vi "OUTPUT(Advanced).vi"(8 "Error In":errorcluster, 11 "VISA resource name":refnum<visa-resource-name>) -> (0 "Error Out":errorcluster, 3 "VISA resource name out":refnum<visa-resource-name>)   [LabVIEW 2013]
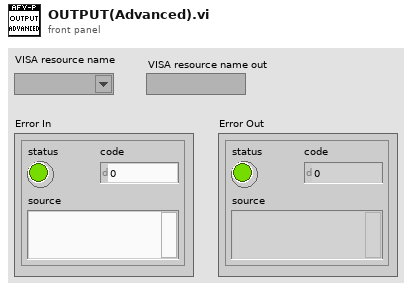
[diagram p1: front panel]
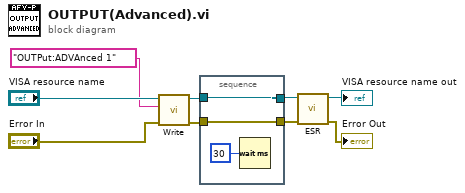
[diagram p0: block diagram]
diagram:
  n1 = call "Write.vi"("Error In"="Error In", "Write Buffer"="OUTPut:ADVAnced 1", "VISA resource name"="VISA resource name") -> ("Error Out"=w1:errorcluster, "VISA resource name out"=w2:refnum<visa-resource-name>)  [unwired: 7 in]
  n2 = stacked-sequence {
    tunnel: [w11] -> w6
    tunnel: w2 -> [w11]
    tunnel: [w10] -> w5
    tunnel: w1 -> [w10]
    frame #0 {
      n3 = Wait (ms)(milliseconds to wait=u32 30) -> ()  [unwired: 1 out]
    }
  }
  n4 = call "ESR.vi"("Error In"=w5, "VISA resource name"=w6) -> ("Error Out"=→"Error Out":errorcluster, "VISA resource name out"=→"VISA resource name out":refnum<visa-resource-name>)  [unwired: 8 in]
